vi "Servo Speed with NI VISA Write .vi"() -> ()   [LabVIEW 2016]
uses:
  <vilib>/Instr/_visa.llb/VISA Configure Serial Port (Instr).vi
panel:
  in  "up":bool
  in  "down":bool
  in  "VISA resource name 3":refnum<visa-resource-name>
  in  "VISA resource name 2":refnum<visa-resource-name>
  in  "STOP":bool
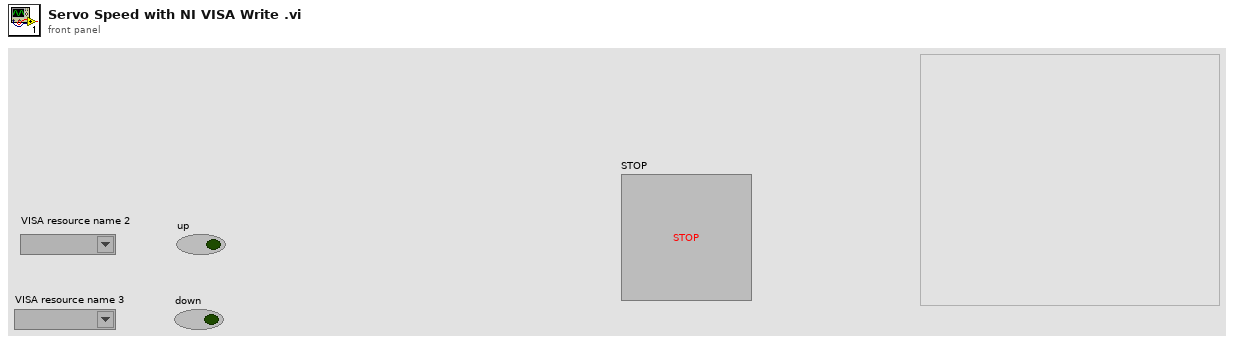
[diagram p1: front panel]
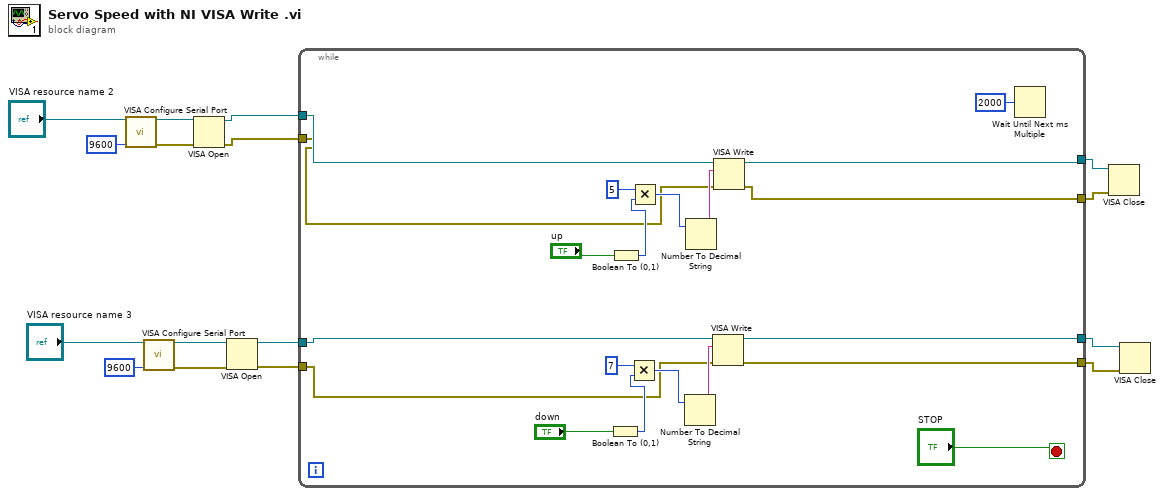
[diagram p0: block diagram]
diagram:
  n1 = call-poly "VISA Configure Serial Port"("VISA resource name"="VISA resource name 2", "baud rate (9600)"=u32 9600) -> ("VISA resource name out"=w13:refnum<visa-resource-name>, "error out"=w10:errorcluster)  [unwired: 12 in]
  n2 = call-poly "VISA Configure Serial Port"("VISA resource name"="VISA resource name 3", "baud rate (9600)"=u32 9600) -> ("VISA resource name out"=w6:refnum<visa-resource-name>, "error out"=w5:errorcluster)  [unwired: 12 in]
  n3 = VISA Open(error in (no error)=w10, VISA resource name=w13) -> (VISA resource name=w12:refnum<visa-resource-name>, error out=w11:errorcluster)  [unwired: 3 in]
  n4 = VISA Open(error in (no error)=w5, VISA resource name=w6) -> (VISA resource name=w4:refnum<visa-resource-name>, error out=w3:errorcluster)  [unwired: 3 in]
  n5 = while {
    tunnel: [w29] -> w16
    tunnel: [w28] -> w15
    tunnel: w12 -> [w31]
    tunnel: w11 -> [w30]
    tunnel: w4 -> [w22]
    tunnel: w3 -> [w21]
    tunnel: [w20] -> w2
    tunnel: [w19] -> w1
    stop <- "STOP" stop-if-true
    n6 = Boolean To (0,1)(Boolean="down") -> (0, 1=w25:i16)
    n7 = Boolean To (0,1)(Boolean="up") -> (0, 1=w33:i16)
    n8 = Multiply(x=i16 7, y=w25) -> (x*y=w26:i16)
    n9 = Multiply(x=i16 5, y=w33) -> (x*y=w34:i16)
    n10 = Number To Decimal String(number=w26) -> (decimal integer string=w24:string)  [unwired: 1 in]
    n11 = Number To Decimal String(number=w34) -> (decimal integer string=w32:string)  [unwired: 1 in]
    n12 = VISA Write(VISA resource name=w22, write buffer=w24, error in (no error)=w21) -> (VISA resource name out=w20:refnum<visa-resource-name>, error out=w19:errorcluster)  [unwired: 1 out]
    n13 = VISA Write(VISA resource name=w31, write buffer=w32, error in (no error)=w30) -> (VISA resource name out=w29:refnum<visa-resource-name>, error out=w28:errorcluster)  [unwired: 1 out]
    n14 = Wait Until Next ms Multiple(millisecond multiple=u32 2000) -> ()  [unwired: 1 out]
  }
  n15 = VISA Close(VISA resource name=w16, error in (no error)=w15) -> ()  [unwired: 1 out]
  n16 = VISA Close(VISA resource name=w2, error in (no error)=w1) -> ()  [unwired: 1 out]
